vi "number of occurance.vi"() -> ()   [LabVIEW 2013]
panel:
  out "Numeric":dbl
  in  "enter the word":string
  in  "Array":string[](array[string])
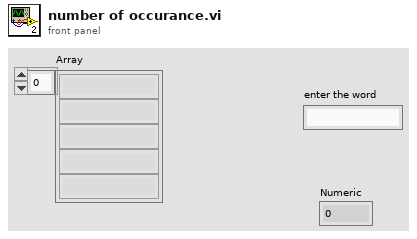
[diagram p1: front panel]
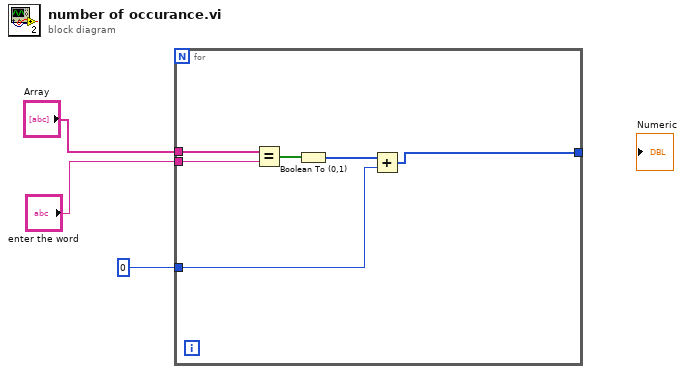
[diagram p0: block diagram]
diagram:
  n1 = for {
    tunnel: "Array" -> [w9]
    tunnel: "enter the word" -> [w8]
    tunnel: [w5] -> _
    tunnel: 0 -> [w4]
    n2 = Equal?(x=w9, y=w8) -> (x = y?=w7:bool[])
    n3 = Boolean To (0,1)(Boolean=w7) -> (0, 1=w6:i16[])
    n4 = Add(x=w6, y=w4) -> (x+y=w5:i32[])
  }
